vi "Persistent Data.vi"(1 "Input":string, 2 "Persistent Data FGV Selector":T2, 3 "Action":T1) -> (0 "Output":string)   [LabVIEW 2013]
uses:
  Persistent Data FGV Selector.ctl
  Action.ctl
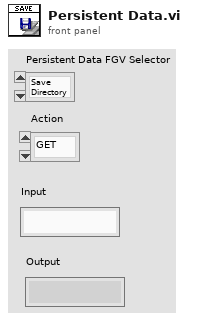
[diagram p1: front panel]
types:
  T1 = typedef "Action.ctl" = enum16{"GET", "PUT", "DELETE"}
  T2 = typedef "Persistent Data FGV Selector.ctl" = enum16{"Save Directory", "File Name"}
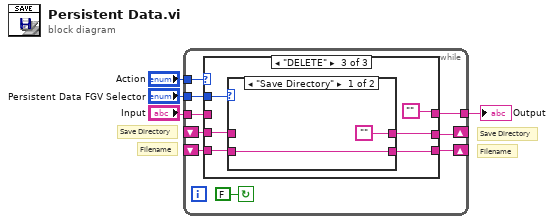
[diagram p0: block diagram]
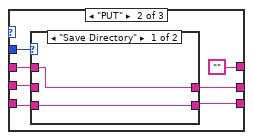
[diagram p4: hidden frame]
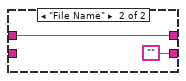
[diagram p6: hidden frame]
diagram:
  # "Filename"
  # "Save Directory"
  # "Filename"
  # "Save Directory"
  n1 = while {
    tunnel: "Input" -> [w6]
    tunnel: "Action" -> [w12]
    tunnel: "Persistent Data FGV Selector" -> [w11]
    shift-right: [w5] -> _
    shift-left: _ -> [w9]
    shift-right: [w8] -> _
    shift-left: _ -> [w7]
    tunnel: [w10] -> w1
    stop <- FALSE continue-if-true
    n2 = case shown="\"DELETE\"" w12 {
      tunnel: w11 -> [w19 w25 w40]
      tunnel: [w15 "" ""] -> w10
      tunnel: w9 -> [w18 w30 w39]
      tunnel: [w17 w27 w36] -> w8
      tunnel: w7 -> [w16 w29 w38]
      tunnel: [w14 w28 w37] -> w5
      tunnel: w6 -> [_ w24 _]
      frame "GET", Default {
        n3 = case shown="\"File Name\"" w19 {
          tunnel: w18 -> [w20 w23]
          tunnel: [w20 w23] -> w14
          tunnel: [w21 w22] -> w17
          tunnel: w16 -> [w21 w22]
          tunnel: [w20 w22] -> w15
          frame "Save Directory" {
          }
          frame "File Name" {
          }
        }
      }
      frame "PUT" {
        n4 = case shown="\"Save Directory\"" w25 {
          tunnel: w30 -> [_ w34]
          tunnel: [w31 w34] -> w28
          tunnel: [w32 w33] -> w27
          tunnel: w29 -> [w32 _]
          tunnel: w24 -> [w31 w33]
          frame "Save Directory" {
          }
          frame "File Name" {
          }
        }
      }
      frame "DELETE" {
        n5 = case shown="\"Save Directory\"" w40 {
          tunnel: w39 -> [_ w44]
          tunnel: ["" w44] -> w37
          tunnel: [w42 ""] -> w36
          tunnel: w38 -> [w42 _]
          frame "Save Directory" {
          }
          frame "File Name" {
          }
        }
      }
    }
  }
  "Output" <- w1
